vi "LockinDAQ.Calibrate.vi"(8 "error in (no error)":errorcluster, 11 "LockinDAQ":refnum<class "LockinDAQ.lvclass">) -> (0 "error out":errorcluster, 2 "Cal Info":T1[](array[typedef]) {"SelfCal.LastDate/Time" format="%<%I:%M %p\n%m/%d/%Y>T"}, 3 "LockinDAQ out":refnum<class "LockinDAQ.lvclass">)   [LabVIEW 2016, in "LockinDAQ.lvclass"]
uses:
  LockinDAQ.lvclass
  Typedefs/Cal Info - Cluster.ctl
  LockinDAQ.lvclass/LockinDAQ.ctl
  <vilib>/addons/WireFlow/_WF_ProgressBar.llb/WindowBehavior.ctl
  <userlib>/_OpenG.lib/array/array.llb/Remove Duplicates from 1D Array (String)__ogtk.vi
  <vilib>/addons/WireFlow/_WF_ProgressBar.llb/ProgressBar_WireFlow.lvclass
  <resource>/objmgr/daqmx.rc
panel:
  out "Numeric":i32
  out "dev temp >5°C from cal temp":bool
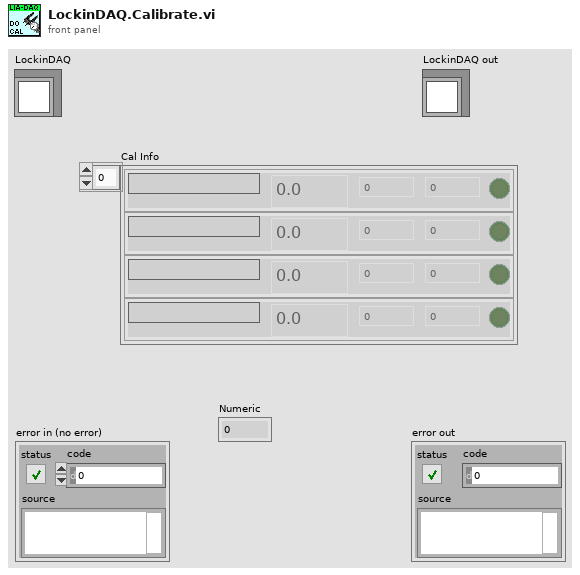
[diagram p1: front panel]
types:
  T1 = typedef "LockinDAQ.lvclass/Cal Info - Cluster.ctl" = cluster{"Active Device":string, "SelfCal.LastDate/Time":dbl, "SelfCal.LastTemp":dbl, "DevTemp":dbl, "calibration due?":bool}
  T2 = typedef "ProgressBar_WireFlow.lvclass/WindowBehavior.ctl" = enum16{"No change", "Modal", "Floating"}
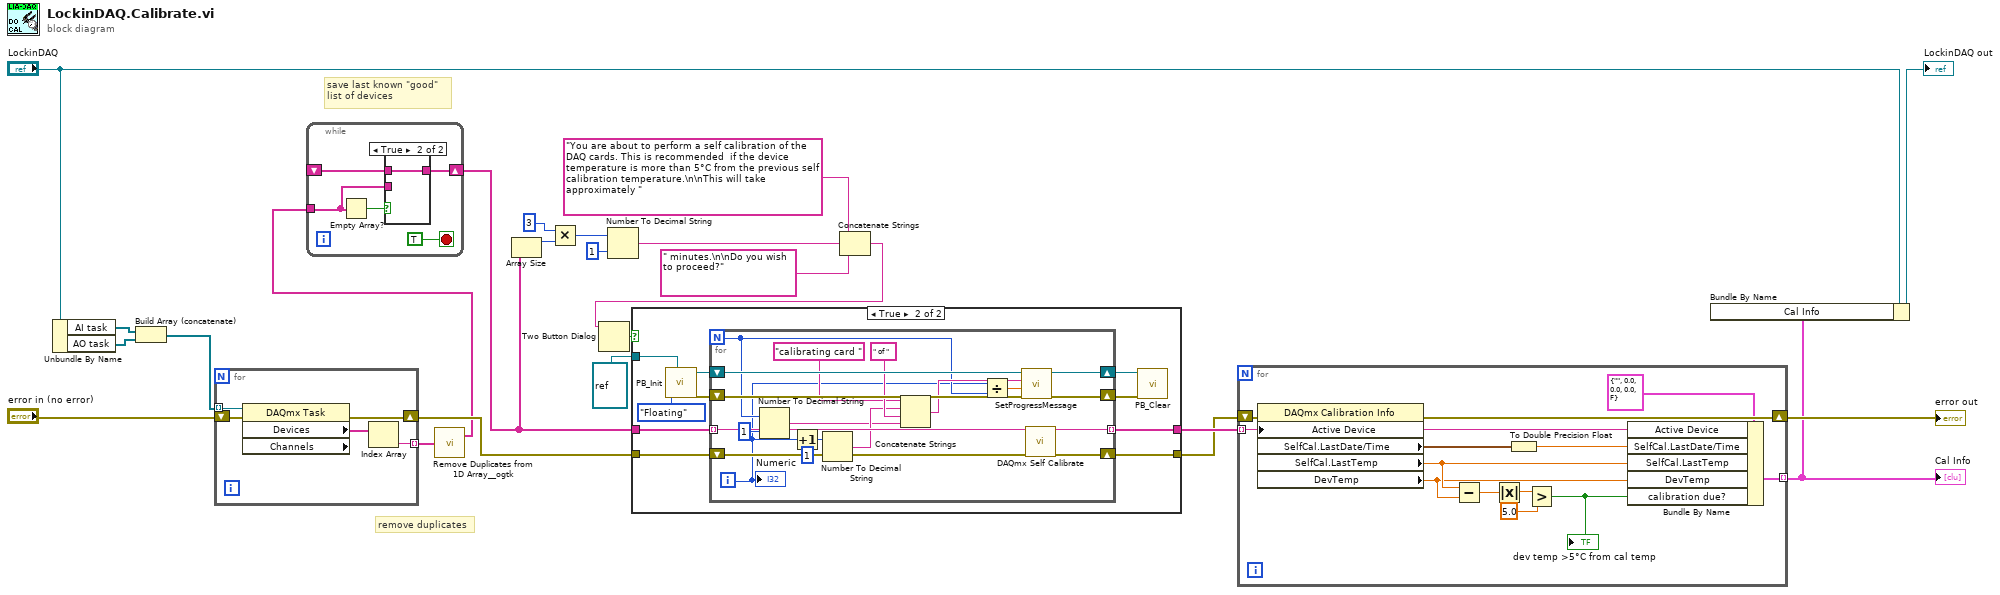
[diagram p0: block diagram]
diagram:
  # "save last known \"good\"\nlist of devices"
  # "remove duplicates"
  n1 = Unbundle By Name("LockinDAQ") -> ("AI task"=w15:refnum<k21>[], "AO task"=w14:refnum<k21>[])
  n2 = Build Array (concatenate)(w15, w14) -> (w23:refnum<k21>[])
  n3 = for {
    tunnel: [w27] -> w22 mode=indexing
    shift-right: [w28] -> w20
    shift-left: "error in (no error)" -> [w29]
    tunnel: w23 -> [w25] mode=indexing
    n4 = property class="DAQmx Task" props=["Devices", "Channels"](reference=w25, error in=w29) -> (error out=w28:errorcluster, "Devices"=w26:tag[])  [unwired: 2 out]
    n5 = Index Array(array=w26) -> (element=w27:tag)  [unwired: 1 in]
  }
  n6 = call-poly <userlib>:"Remove Duplicates from 1D Array__ogtk.vi"("Input Array"=w22) -> ("Output Array"=w17:string[])  [unwired: 1 out]
  n7 = while {
    shift-right: [w32] -> w16
    shift-left: _ -> [w30]
    tunnel: w17 -> [w31]
    stop <- TRUE stop-if-true
    n8 = Empty Array?(array=w31) -> (empty?=w33:bool)
    n9 = case shown="True" w33 {
      tunnel: [w35 w36] -> w32
      tunnel: w31 -> [w35 _]
      tunnel: w30 -> [_ w36]
      frame False {
      }
      frame True {
      }
    }
  }
  n10 = Array Size(array=w16) -> (size(s)=w11:i32)
  n11 = Multiply(x=3, y=w11) -> (x*y=w3:i32)
  n12 = Number To Decimal String(number=w3, width (-)=i16 1) -> (decimal integer string=w4:string)
  n13 = Concatenate Strings("You are about to perform a self calibration of the DAQ cards. This is recommended  if the device temperature is more than 5°C from the previous self calibration temperature.\n\nThis will take approximately " ("message"), w4, " minutes.\n\nDo you wish to proceed?") -> (w5:string)
  n14 = Two Button Dialog(message=w5) -> (T button?=w6:bool)  [unwired: 2 in]
  n15 = case shown="True" w6 {
    tunnel: w20 -> [w38 w48]
    tunnel: [w38 w47] -> w18
    tunnel: [w37 w46] -> w19
    tunnel: w16 -> [w37 w45]
    tunnel: refnum<vi> refnum ("Progress VI") -> [_ w40]
    frame False {
    }
    frame True {
      n16 = call <vilib>:"PB_Init.vi"("Progress VI"=w40, "Window behavior (No change)"=WindowBehavior."Floating") -> ("error out"=w41:errorcluster, "WF-ProgressBar out"=w42:refnum<class "ProgressBar_WireFlow.lvclass">)  [unwired: 8 in]
      n17 = for {
        N -> [w55]
        shift-right: [w65] -> w47
        shift-left: w48 -> [w66]
        tunnel: w45 -> [w64] mode=indexing
        tunnel: [w64] -> w46 mode=indexing
        shift-right: [w61] -> w44
        shift-left: w42 -> [w62]
        shift-right: [w60] -> w43
        shift-left: w41 -> [w63]
        i -> [w50]
        n18 = Number To Decimal String(number=w55, width (-)=i16 1) -> (decimal integer string=w51:string)
        n19 = Increment(x=w50) -> (x+1=w49:i32)
        n20 = Number To Decimal String(number=w49, width (-)=i16 1) -> (decimal integer string=w53:string)
        n21 = Concatenate Strings("calibrating card ", w53, " of ", w51) -> (w56:string)
        n22 = Divide(x=w50, y=w55) -> (x/y=w57:dbl)
        n23 = call-dynamic "SetProgressMessage.vi"("error in (no error)"=w63, "Progress value (NaN no update)"=w57, "Message"=w56, "WF-ProgressBar in"=w62) -> ("error out"=w60:errorcluster, "WF-ProgressBar out"=w61:refnum<class "ProgressBar_WireFlow.lvclass">)  [unwired: 5 in, 1 out]
        n24 = call <vilib>:"DAQmx Self Calibrate.vi"("device in"=w64, "error in"=w66) -> ("error out"=w65:errorcluster)  [unwired: 13 in]
        "Numeric" <- w50
      }
      n25 = call-dynamic "PB_Clear.vi"("error in (no error)"=w43, "WF-ProgressBar in"=w44) -> ()  [unwired: 8 in, 2 out]
    }
  }
  n26 = for {
    tunnel: [w78] -> w1 mode=indexing
    shift-right: [w79] -> w21
    shift-left: w18 -> [w77]
    tunnel: w19 -> [w72] mode=indexing
    n27 = property class="DAQmx Calibration Info"(error in=w77, "Active Device"=w72) -> (error out=w79:errorcluster, "SelfCal.LastDate/Time"=w68:timestamp, "SelfCal.LastTemp"=w70:dbl, "DevTemp"=w69:dbl)  [unwired: 1 in, 1 out]
    n28 = Subtract(x=w70, y=w69) -> (x-y=w76:dbl)
    n29 = Absolute Value(x=w76) -> (abs(x)=w75:dbl)
    n30 = To Double Precision Float(number=w68) -> (double precision float=w67:dbl)
    n31 = Greater?(x=w75, y=5.0) -> (0:w73:bool)
    "dev temp >5°C from cal temp" <- w73
    n32 = Bundle By Name(cluster=T1 {"Active Device"="", "SelfCal.LastDate/Time"=0.0, "SelfCal.LastTemp"=0.0, "DevTemp"=0.0, "calibration due?"=FALSE} ("Calibration"), "Active Device"=w72, "SelfCal.LastDate/Time"=w67, "SelfCal.LastTemp"=w70, "DevTemp"=w69, "calibration due?"=w73) -> (w78:T1)
  }
  "error out" <- w21
  "Cal Info" <- w1
  n33 = Bundle By Name(cluster="LockinDAQ", "Cal Info"=w1) -> (→"LockinDAQ out":refnum<class "LockinDAQ.lvclass">)
